vi "Image Zoom-in.vi"(8 "error in (no error)":errorcluster, 9 "Target Corners":T1, 10 "Original":T2, 11 "Processed":T2) -> (0 "error out":errorcluster, 3 "Processed out":T2)   [LabVIEW 2011]
uses:
  <vilib>/vision/Image Controls.llb/IMAQ Image.ctl
  <vilib>/vision/NI_Vision_Development_Module.lvlib
panel:
  out "Array 2":cluster{i32, i32}[](array[cluster])
  out "Array":cluster{i32, i32}[](array[cluster])
  out "Original":T2(plugin-control)
  out "Processed":T2(plugin-control)
  out "32bit integer":i32[](array[numeric])
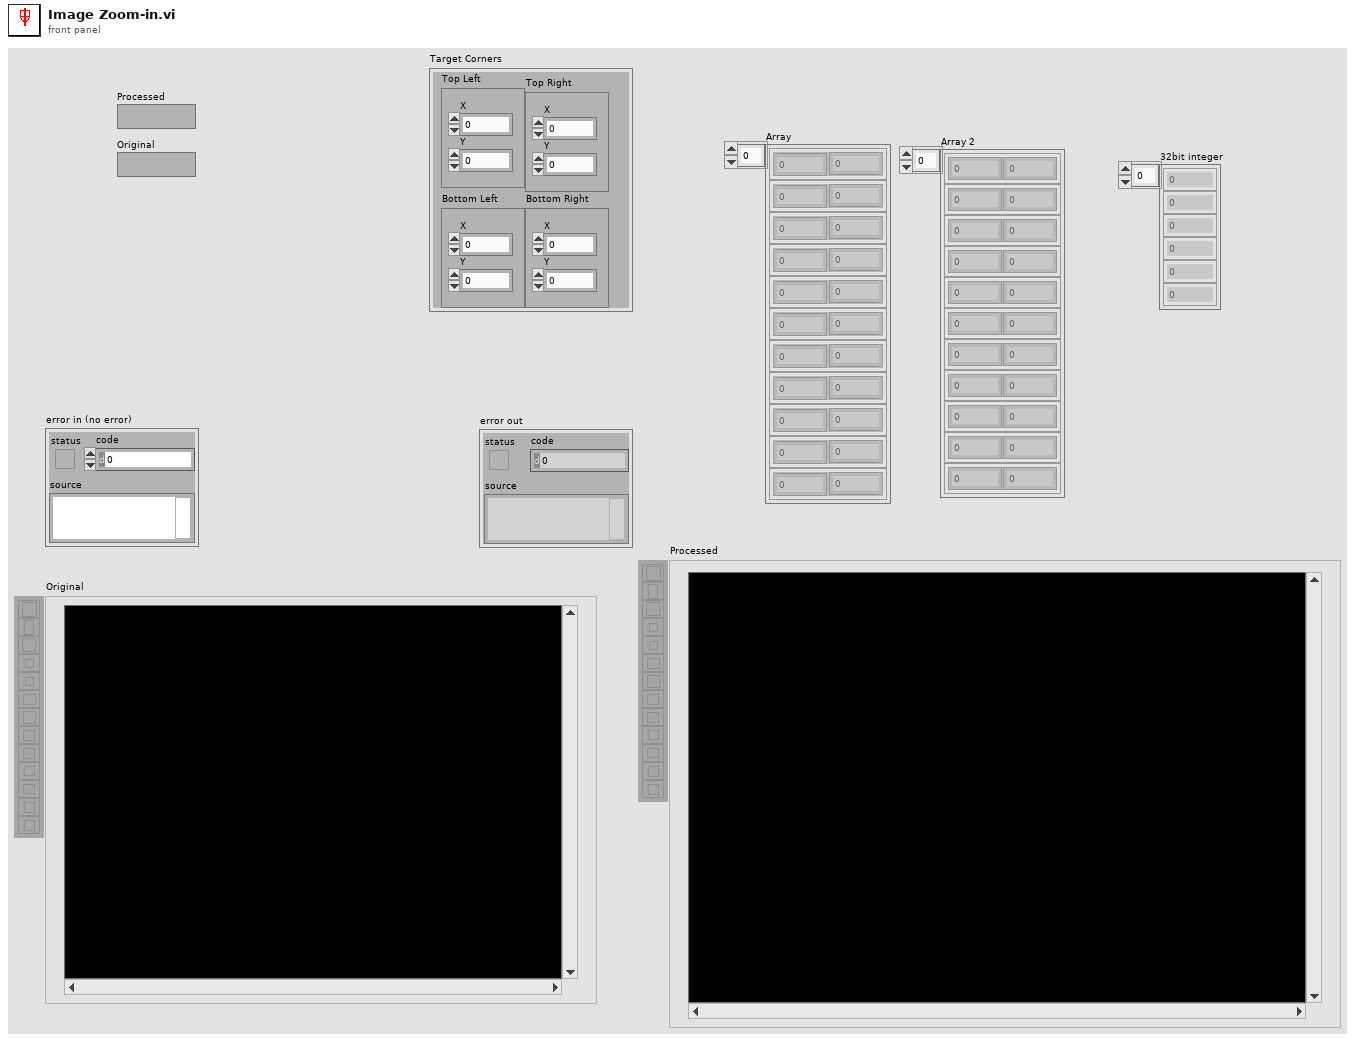
[diagram p1: front panel]
types:
  T1 = cluster{"Bottom Left":cluster{"X":dbl, "Y":dbl}, "Bottom Right":cluster{"X":dbl, "Y":dbl}, "Top Right":cluster{"X":dbl, "Y":dbl}, "Top Left":cluster{"X":dbl, "Y":dbl}}
  T2 = typedef "IMAQ Image.ctl" = refnum<image>
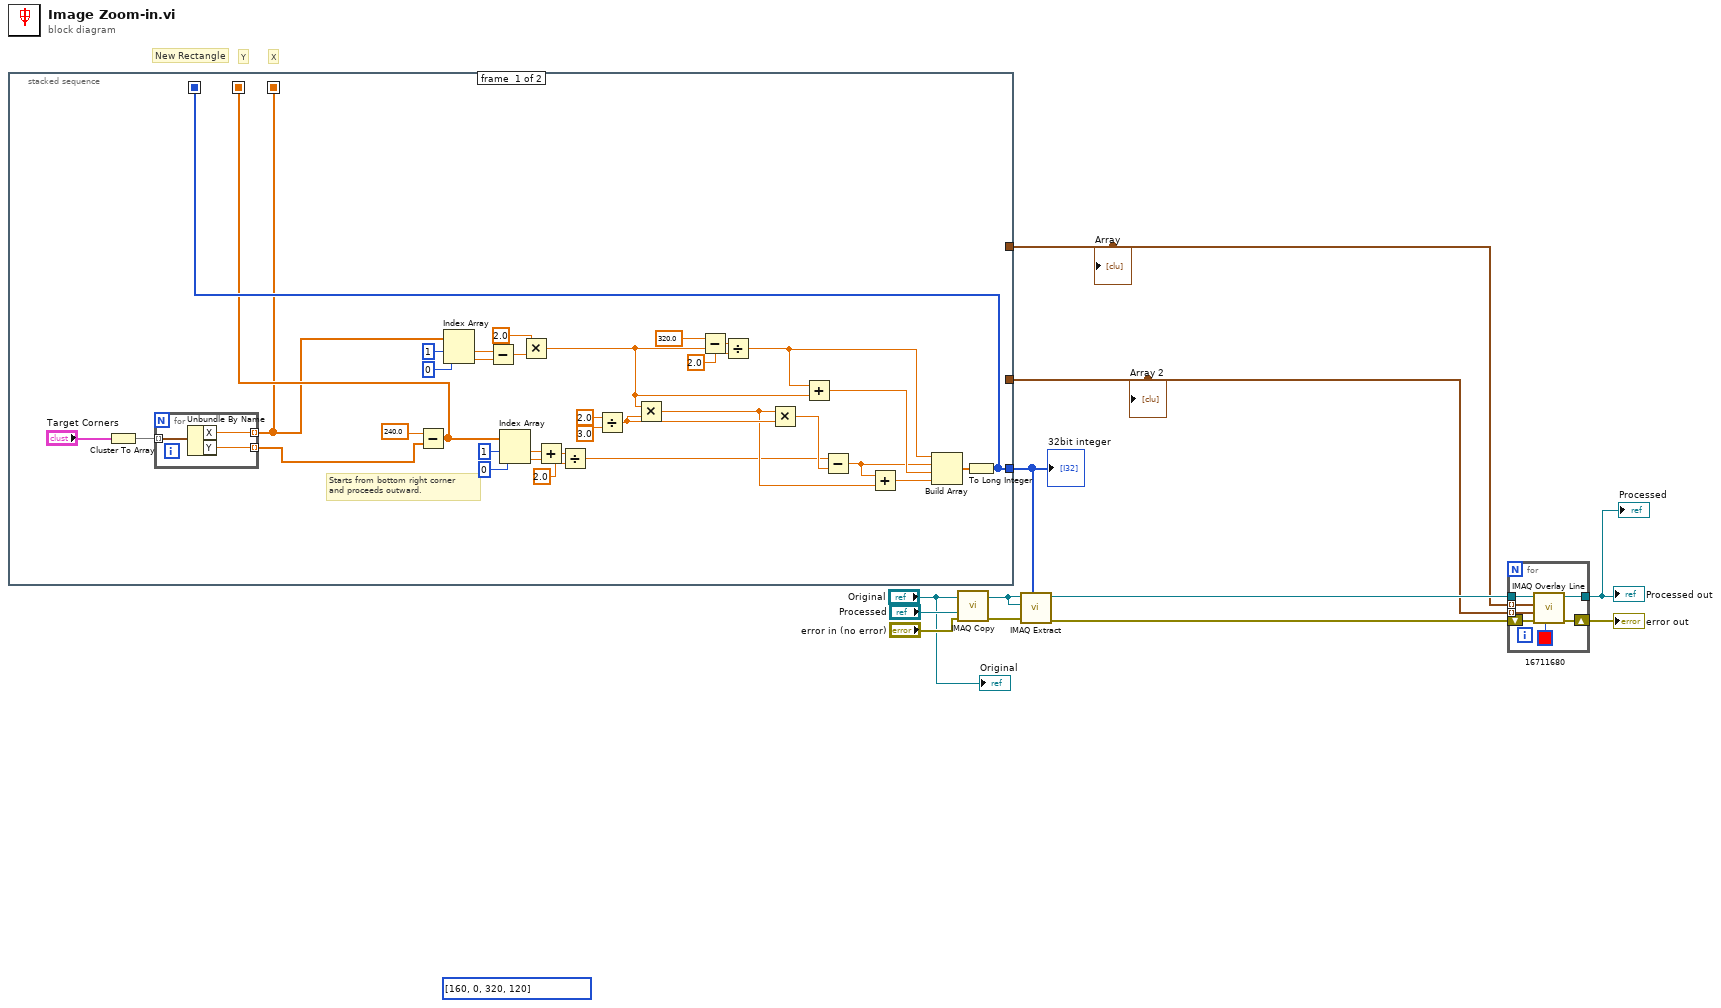
[diagram p0: block diagram]
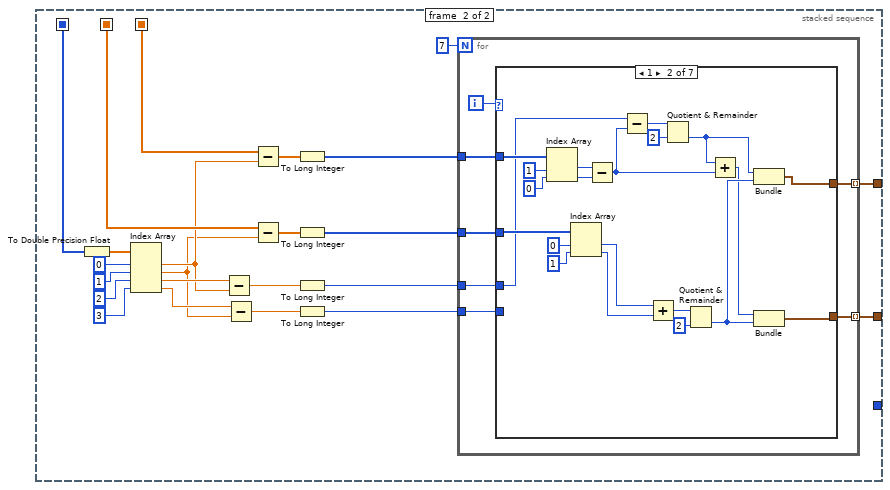
[diagram p2: hidden frame]
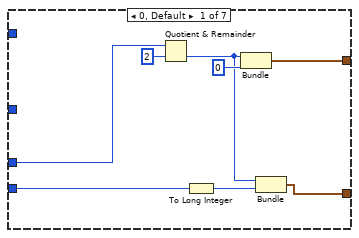
[diagram p3: hidden frame]
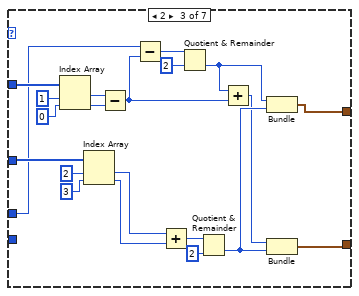
[diagram p4: hidden frame]
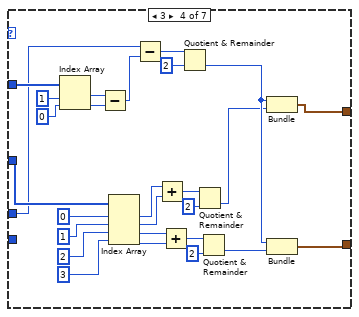
[diagram p5: hidden frame]
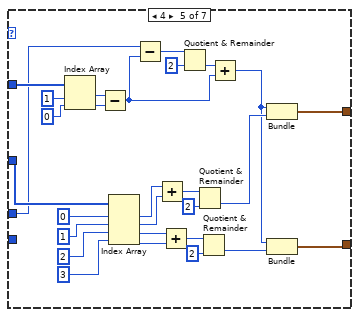
[diagram p6: hidden frame]
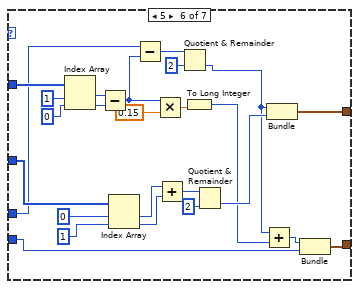
[diagram p7: hidden frame]
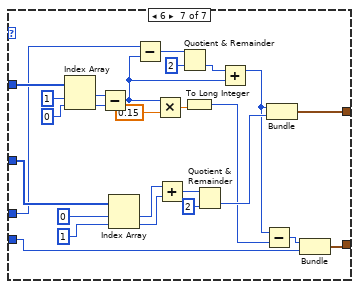
[diagram p8: hidden frame]
diagram:
  (unwired) i32[] [160, 0, 320, 120] ("Optional Rectangle")
  # "Y"
  # "X"
  # "New Rectangle"
  n1 = stacked-sequence {
    seq-local: [w14 _] -> [_ w69]
    seq-local: [w17 _] -> [_ w68]
    seq-local: [w18 _] -> [_ w72]
    tunnel: [w18 _] -> w6
    tunnel: [_ w57] -> w2
    tunnel: [_ w55] -> w1
    frame #0 {
      # "Starts from bottom right corner\nand proceeds outward."
      n2 = Cluster To Array(cluster="Target Corners") -> (array=w15:cluster{"X":dbl, "Y":dbl}[])
      n3 = for {
        tunnel: w15 -> [w49] mode=indexing
        tunnel: [w48] -> w14 mode=indexing
        tunnel: [w47] -> w13 mode=indexing
        n4 = Unbundle By Name(w49) -> ("X"=w48:dbl, "Y"=w47:dbl)
      }
      n5 = Subtract(x=240.0, y=w13) -> (x-y=w17:dbl[])
      n6 = Index Array(array=w14, index #1=1 ("index"), index #2=0 ("index")) -> (element #1=w43:dbl, element #2=w44:dbl)
      n7 = Subtract(x=w43, y=w44) -> (x-y=w42:dbl)
      n8 = Index Array(array=w17, index #1=1 ("index"), index #2=0 ("index")) -> (element #1=w34:dbl, element #2=w35:dbl)
      n9 = Multiply(x=2.0, y=w42) -> (x*y=w26:dbl)
      n10 = Add(x=w34, y=w35) -> (x+y=w33:dbl)
      n11 = Divide(x=w33, y=2.0) -> (x/y=w20:dbl)
      n12 = Divide(x=2.0, y=3.0) -> (x/y=w29:dbl)
      n13 = Multiply(x=w26, y=w29) -> (x*y=w23:dbl)
      n14 = Subtract(x=320.0, y=w26) -> (x-y=w39:dbl)
      n15 = Divide(x=w39, y=2.0) -> (x/y=w27:dbl)
      n16 = Multiply(x=w23, y=w29) -> (x*y=w28:dbl)
      n17 = Add(x=w27, y=w26) -> (x+y=w25:dbl)
      n18 = Subtract(x=w20, y=w28) -> (x-y=w24:dbl)
      n19 = Add(x=w24, y=w23) -> (x+y=w22:dbl)
      n20 = Build Array(w27, w24, w25, w22) -> (w21:dbl[])
      n21 = To Long Integer(number=w21) -> (32bit integer=w18:i32[])
    }
    frame #1 {
      n22 = To Double Precision Float(number=w72) -> (double precision float=w67:dbl[])
      n23 = Index Array(array=w67, index #1=0 ("index"), index #2=1 ("index"), index #3=2 ("index"), index #4=3 ("index")) -> (element #1=w63:dbl, element #2=w50:dbl, element #3=w64:dbl, element #4=w61:dbl)
      n24 = Subtract(x=w64, y=w63) -> (x-y=w62:dbl)
      n25 = Subtract(x=w61, y=w50) -> (x-y=w60:dbl)
      n26 = Subtract(x=w69, y=w63) -> (x-y=w54:dbl[])
      n27 = Subtract(x=w68, y=w50) -> (x-y=w53:dbl[])
      n28 = To Long Integer(number=w54) -> (32bit integer=w52:i32[])
      n29 = To Long Integer(number=w53) -> (32bit integer=w51:i32[])
      n30 = To Long Integer(number=w62) -> (32bit integer=w59:i32)
      n31 = To Long Integer(number=w60) -> (32bit integer=w58:i32)
      n32 = for {
        N: 7 -> [_]
        tunnel: w52 -> [w76]
        tunnel: w51 -> [w75]
        tunnel: w59 -> [w78]
        tunnel: w58 -> [w77]
        tunnel: [w74] -> w57 mode=indexing
        tunnel: [w73] -> w55 mode=indexing
        i -> [w79]
        n33 = case shown="1" w79 {
          tunnel: w78 -> [w81 w90 w111 w139 w167 w199 w225]
          tunnel: w77 -> [w87 _ _ _ _ w191 w217]
          tunnel: w76 -> [_ w106 w127 w154 w182 w207 w233]
          tunnel: w75 -> [_ w103 w124 w151 w179 w206 w232]
          tunnel: [w84 w102 w123 w150 w178 w205 w231] -> w74
          tunnel: [w83 w101 w122 w149 w177 w204 w230] -> w73
          frame 0, Default {
            n34 = Quotient & Remainder(x=w81, y=2) -> (floor(x/y)=w80:i32)  [unwired: 1 out]
            n35 = To Long Integer(number=w87) -> (32bit integer=w85:i32)
            n36 = Bundle(w80, 0) -> (w84:cluster{i32, i32})  [unwired: 1 in]
            n37 = Bundle(w80, w85) -> (w83:cluster{i32, i32})  [unwired: 1 in]
          }
          frame 1 {
            n38 = Index Array(array=w106, index #1=1 ("index"), index #2=0 ("index")) -> (element #1=w93:i32, element #2=w92:i32)
            n39 = Index Array(array=w103, index #1=0 ("index"), index #2=1 ("index")) -> (element #1=w100:i32, element #2=w99:i32)
            n40 = Subtract(x=w93, y=w92) -> (x-y=w89:i32)
            n41 = Subtract(x=w90, y=w89) -> (x-y=w91:i32)
            n42 = Add(x=w100, y=w99) -> (x+y=w98:i32)
            n43 = Quotient & Remainder(x=w91, y=2) -> (floor(x/y)=w88:i32)  [unwired: 1 out]
            n44 = Quotient & Remainder(x=w98, y=2) -> (floor(x/y)=w96:i32)  [unwired: 1 out]
            n45 = Add(x=w88, y=w89) -> (x+y=w94:i32)
            n46 = Bundle(w88, w96) -> (w102:cluster{i32, i32})  [unwired: 1 in]
            n47 = Bundle(w94, w96) -> (w101:cluster{i32, i32})  [unwired: 1 in]
          }
          frame 2 {
            n48 = Index Array(array=w127, index #1=1 ("index"), index #2=0 ("index")) -> (element #1=w114:i32, element #2=w113:i32)
            n49 = Index Array(array=w124, index #1=2 ("index"), index #2=3 ("index")) -> (element #1=w121:i32, element #2=w120:i32)
            n50 = Subtract(x=w114, y=w113) -> (x-y=w110:i32)
            n51 = Subtract(x=w111, y=w110) -> (x-y=w112:i32)
            n52 = Add(x=w121, y=w120) -> (x+y=w119:i32)
            n53 = Quotient & Remainder(x=w112, y=2) -> (floor(x/y)=w109:i32)  [unwired: 1 out]
            n54 = Quotient & Remainder(x=w119, y=2) -> (floor(x/y)=w117:i32)  [unwired: 1 out]
            n55 = Add(x=w109, y=w110) -> (x+y=w115:i32)
            n56 = Bundle(w109, w117) -> (w123:cluster{i32, i32})  [unwired: 1 in]
            n57 = Bundle(w115, w117) -> (w122:cluster{i32, i32})  [unwired: 1 in]
          }
          frame 3 {
            n58 = Index Array(array=w154, index #1=1 ("index"), index #2=0 ("index")) -> (element #1=w142:i32, element #2=w141:i32)
            n59 = Subtract(x=w142, y=w141) -> (x-y=w138:i32)
            n60 = Index Array(array=w151, index #1=0 ("index"), index #2=1 ("index"), index #3=2 ("index"), index #4=3 ("index")) -> (element #1=w132:i32, element #2=w131:i32, element #3=w148:i32, element #4=w147:i32)
            n61 = Subtract(x=w139, y=w138) -> (x-y=w140:i32)
            n62 = Add(x=w132, y=w131) -> (x+y=w133:i32)
            n63 = Add(x=w148, y=w147) -> (x+y=w146:i32)
            n64 = Quotient & Remainder(x=w140, y=2) -> (floor(x/y)=w137:i32)  [unwired: 1 out]
            n65 = Quotient & Remainder(x=w133, y=2) -> (floor(x/y)=w130:i32)  [unwired: 1 out]
            n66 = Quotient & Remainder(x=w146, y=2) -> (floor(x/y)=w144:i32)  [unwired: 1 out]
            n67 = Bundle(w137, w130) -> (w150:cluster{i32, i32})  [unwired: 1 in]
            n68 = Bundle(w137, w144) -> (w149:cluster{i32, i32})  [unwired: 1 in]
          }
          frame 4 {
            n69 = Index Array(array=w182, index #1=1 ("index"), index #2=0 ("index")) -> (element #1=w170:i32, element #2=w169:i32)
            n70 = Subtract(x=w170, y=w169) -> (x-y=w158:i32)
            n71 = Index Array(array=w179, index #1=0 ("index"), index #2=1 ("index"), index #3=2 ("index"), index #4=3 ("index")) -> (element #1=w161:i32, element #2=w160:i32, element #3=w176:i32, element #4=w175:i32)
            n72 = Subtract(x=w167, y=w158) -> (x-y=w168:i32)
            n73 = Add(x=w161, y=w160) -> (x+y=w162:i32)
            n74 = Add(x=w176, y=w175) -> (x+y=w174:i32)
            n75 = Quotient & Remainder(x=w168, y=2) -> (floor(x/y)=w166:i32)  [unwired: 1 out]
            n76 = Quotient & Remainder(x=w162, y=2) -> (floor(x/y)=w159:i32)  [unwired: 1 out]
            n77 = Quotient & Remainder(x=w174, y=2) -> (floor(x/y)=w172:i32)  [unwired: 1 out]
            n78 = Add(x=w166, y=w158) -> (x+y=w157:i32)
            n79 = Bundle(w157, w159) -> (w178:cluster{i32, i32})  [unwired: 1 in]
            n80 = Bundle(w157, w172) -> (w177:cluster{i32, i32})  [unwired: 1 in]
          }
          frame 5 {
            n81 = Index Array(array=w207, index #1=1 ("index"), index #2=0 ("index")) -> (element #1=w202:i32, element #2=w201:i32)
            n82 = Subtract(x=w202, y=w201) -> (x-y=w188:i32)
            n83 = Index Array(array=w206, index #1=0 ("index"), index #2=1 ("index")) -> (element #1=w194:i32, element #2=w193:i32)
            n84 = Subtract(x=w199, y=w188) -> (x-y=w200:i32)
            n85 = Multiply(x=w188, y=0.15) -> (x*y=w186:dbl)
            n86 = Add(x=w194, y=w193) -> (x+y=w195:i32)
            n87 = Quotient & Remainder(x=w200, y=2) -> (floor(x/y)=w189:i32)  [unwired: 1 out]
            n88 = To Long Integer(number=w186) -> (32bit integer=w185:i32)
            n89 = Quotient & Remainder(x=w195, y=2) -> (floor(x/y)=w192:i32)  [unwired: 1 out]
            n90 = Add(x=w189, y=w185) -> (x+y=w190:i32)
            n91 = Bundle(w189, w192) -> (w205:cluster{i32, i32})  [unwired: 1 in]
            n92 = Bundle(w190, w191) -> (w204:cluster{i32, i32})  [unwired: 1 in]
          }
          frame 6 {
            n93 = Index Array(array=w233, index #1=1 ("index"), index #2=0 ("index")) -> (element #1=w228:i32, element #2=w227:i32)
            n94 = Subtract(x=w228, y=w227) -> (x-y=w210:i32)
            n95 = Index Array(array=w232, index #1=0 ("index"), index #2=1 ("index")) -> (element #1=w220:i32, element #2=w219:i32)
            n96 = Subtract(x=w225, y=w210) -> (x-y=w226:i32)
            n97 = Multiply(x=w210, y=0.15) -> (x*y=w213:dbl)
            n98 = Add(x=w220, y=w219) -> (x+y=w221:i32)
            n99 = Quotient & Remainder(x=w226, y=2) -> (floor(x/y)=w215:i32)  [unwired: 1 out]
            n100 = To Long Integer(number=w213) -> (32bit integer=w212:i32)
            n101 = Quotient & Remainder(x=w221, y=2) -> (floor(x/y)=w218:i32)  [unwired: 1 out]
            n102 = Add(x=w215, y=w210) -> (x+y=w211:i32)
            n103 = Subtract(x=w211, y=w212) -> (x-y=w216:i32)
            n104 = Bundle(w211, w218) -> (w231:cluster{i32, i32})  [unwired: 1 in]
            n105 = Bundle(w216, w217) -> (w230:cluster{i32, i32})  [unwired: 1 in]
          }
        }
      }
    }
  }
  "32bit integer" <- w6
  "Array" <- w2
  "Array 2" <- w1
  n106 = call "IMAQ Copy"("error in (no error)"="error in (no error)", "Image Dst"="Processed", "Image Src"="Original") -> ("error out"=w9:errorcluster, "Image Dst Out"=w11:T2)  [unwired: 3 in]
  n107 = call "IMAQ Extract"("Optional Rectangle"=w6, "error in (no error)"=w9, "Image Dst"=w11, "Image Src"=w11) -> ("error out"=w8:errorcluster, "Image Dst Out"=w12:T2)  [unwired: 6 in]
  n108 = for {
    tunnel: w12 -> [w241]
    tunnel: [w240] -> w5
    tunnel: w2 -> [w239] mode=indexing
    tunnel: w1 -> [w238] mode=indexing
    shift-right: [w236] -> w7
    shift-left: w8 -> [w237]
    n109 = call "IMAQ Overlay Line"("Color"=u32 16711680, "error in (no error)"=w237, "End Point"=w238, "Start Point"=w239, "Image"=w241) -> ("error out"=w236:errorcluster, "Image Out"=w240:T2)  [unwired: 5 in]
  }
  "Processed out" <- w5
  "error out" <- w7
  "Processed" <- w5
  "Original" <- "Original"
